vi "Disable Selected Opposing Channels.vi"(6 "Disabled? (False)":bool, 7 "Symbol Index (38)":i32=38, 8 "error in (no error)":errorcluster, 9 "Parent":string, 10 "Node Ptr":u64 format="%.0x", 11 "Tree":refnum<vi>) -> (0 "error out":errorcluster, 2 "Node Ptr":u64 format="%.0x", 3 "Tree Out":refnum<vi>)   [LabVIEW 2013, in "J1939 Addon System Explorer.lvlib"]
uses:
  J1939 Addon System Explorer.lvlib
  <vilib>/NI Veristand/Custom Device API/Custom Device API.lvlib
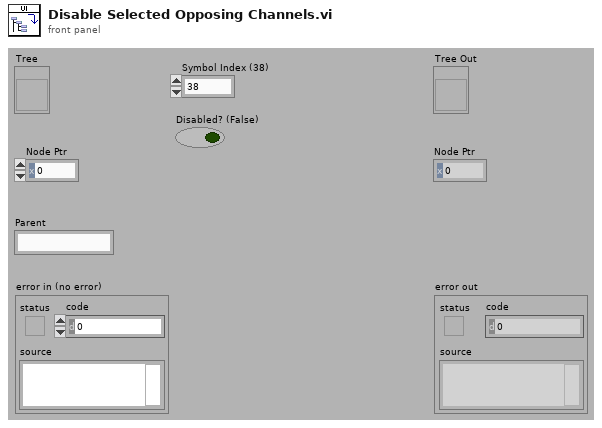
[diagram p1: front panel]
types:
  T1 = typedef "Custom Device API.lvlib/Custom Device Item Ref.ctl" = u64
  T2 = typedef "Custom Device API.lvlib/Custom Device Item Info.ctl" = cluster{"Name":string, "Is Channel":bool, "GUID":string, "Is Waveform":bool}
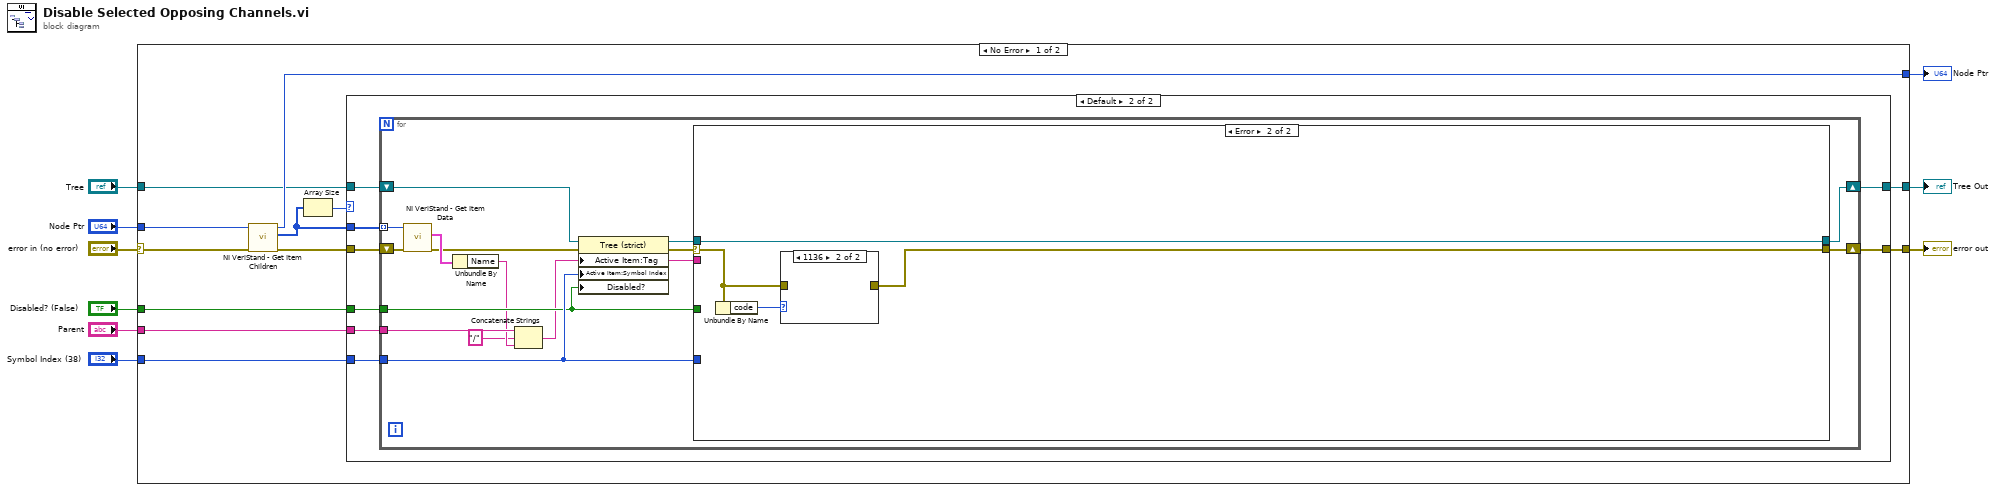
[diagram p0: block diagram]
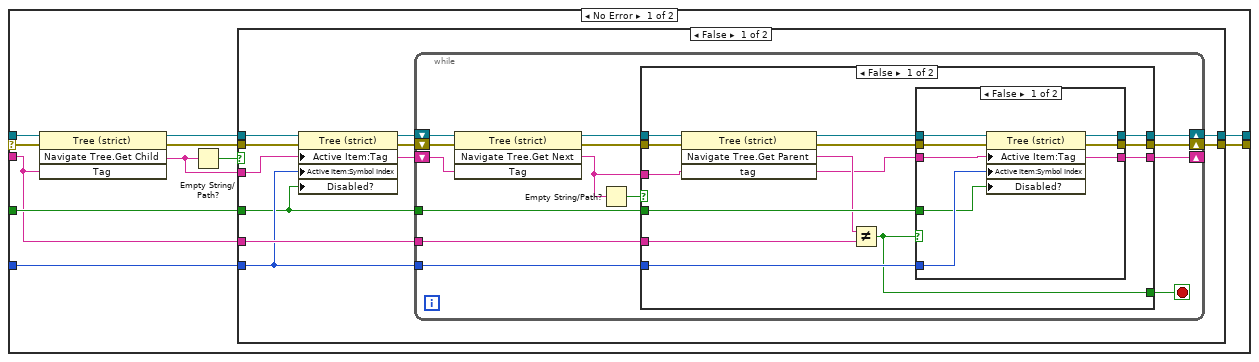
[diagram p3: hidden frame]
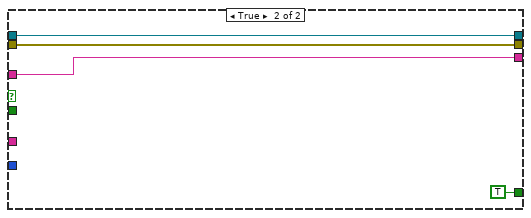
[diagram p5: hidden frame]
diagram:
  n1 = case shown="No Error" "error in (no error)" {
    selector: "error in (no error)" -> [w11 w118]
    tunnel: [w21 w118] -> w8
    tunnel: "Node Ptr" -> [w10 w116]
    tunnel: "Tree" -> [w17 w117]
    tunnel: [w20 w117] -> w5
    tunnel: "Parent" -> [w16 _]
    tunnel: [w19 w116] -> w3
    tunnel: "Symbol Index (38)" -> [w13 _]
    tunnel: "Disabled? (False)" -> [w12 _]
    frame No Error {
      n2 = call <vilib>:"NI VeriStand - Get Item Children.vi"("error in (no error)"=w11, "Item Ref in"=w10) -> ("error out"=w18:errorcluster, "Child Refs"=w15:T1[], "Item Ref out"=w19:T1)  [unwired: 6 in, 1 out]
      n3 = Array Size(array=w15) -> (size(s)=w14:i32)
      n4 = case shown="Default" w14 {
        tunnel: [w23 w31] -> w21
        tunnel: [w22 w30] -> w20
        tunnel: w18 -> [w23 w29]
        tunnel: w17 -> [w22 w28]
        tunnel: w16 -> [_ w26]
        tunnel: w15 -> [_ w25]
        tunnel: w13 -> [_ w24]
        tunnel: w12 -> [_ w27]
        frame 0 {
        }
        frame Default {
          n5 = for {
            tunnel: w25 -> [w45] mode=indexing
            shift-right: [w41] -> w30
            shift-left: w28 -> [w42]
            shift-right: [w40] -> w31
            shift-left: w29 -> [w46]
            tunnel: w26 -> [w39]
            tunnel: w24 -> [w38]
            tunnel: w27 -> [w37]
            n6 = call <vilib>:"NI VeriStand - Get Item Data.vi"("error in (no error)"=w46, "Item Ref in"=w45) -> ("error out"=w43:errorcluster, "Item Info"=w44:T2)  [unwired: 6 in, 2 out]
            n7 = Unbundle By Name(w44) -> ("Name"=w33:string)
            n8 = Concatenate Strings(w39, "/" ("string"), w33) -> (w34:string)
            n9 = property class="Tree (strict)"(reference=w42, error in=w43, "Active Item:Tag"=w34, "Active Item:Symbol Index"=w38, "Disabled?"=w37) -> (reference out=w36:refnum<vi>, error out=w35:errorcluster)
            n10 = case shown="Error" w35 {
              selector: w35 -> [w47 w111]
              tunnel: [w57 w114] -> w41
              tunnel: [w56 w112] -> w40
              tunnel: w38 -> [w55 _]
              tunnel: w37 -> [w54 _]
              tunnel: w34 -> [w53 _]
              tunnel: w36 -> [w52 w114]
              frame No Error {
                n11 = invoke class="Tree (strict)" method="Navigate Tree.Get Child"(reference=w52, error in=w47, "Tag"=w53) -> (reference out=w51:refnum<vi>, error out=w49:errorcluster, "Navigate Tree:Get Child"=w48:string)  [unwired: 1 in, 1 out]
                n12 = Empty String/Path?(string/path=w48) -> (empty?=w50:bool)
                n13 = case shown="False" w50 {
                  tunnel: [w67 w109] -> w57
                  tunnel: [w66 w110] -> w56
                  tunnel: w55 -> [w60 _]
                  tunnel: w54 -> [w59 _]
                  tunnel: w53 -> [w65 _]
                  tunnel: w51 -> [w62 w109]
                  tunnel: w49 -> [w64 w110]
                  tunnel: w48 -> [w58 _]
                  frame False {
                    n14 = property class="Tree (strict)"(reference=w62, error in=w64, "Active Item:Tag"=w58, "Active Item:Symbol Index"=w60, "Disabled?"=w59) -> (reference out=w61:refnum<vi>, error out=w63:errorcluster)
                    n15 = while {
                      shift-right: [w81] -> w67
                      shift-left: w61 -> [w77]
                      shift-right: [w80] -> w66
                      shift-left: w63 -> [w76]
                      tunnel: w65 -> [w72]
                      tunnel: w60 -> [w79]
                      tunnel: w59 -> [w78]
                      shift-right: [w71] -> _
                      shift-left: w58 -> [w75]
                      stop <- w70 stop-if-true
                      n16 = invoke class="Tree (strict)" method="Navigate Tree.Get Next"(reference=w77, error in=w76, "Tag"=w75) -> (reference out=w74:refnum<vi>, error out=w73:errorcluster, "Navigate Tree:Get Next Item"=w69:string)  [unwired: 1 in, 1 out]
                      n17 = Empty String/Path?(string/path=w69) -> (empty?=w68:bool)
                      n18 = case shown="False" w68 {
                        tunnel: [w94 w106] -> w81
                        tunnel: [w93 w107] -> w80
                        tunnel: w79 -> [w92 _]
                        tunnel: w78 -> [w91 _]
                        tunnel: w74 -> [w90 w106]
                        tunnel: w73 -> [w88 w107]
                        tunnel: w72 -> [w86 _]
                        tunnel: [w85 w108] -> w71
                        tunnel: [w84 TRUE] -> w70
                        tunnel: w69 -> [w82 w108]
                        frame False {
                          n19 = invoke class="Tree (strict)" method="Navigate Tree.Get Parent"(reference=w90, error in=w88, "tag"=w82) -> (reference out=w89:refnum<vi>, error out=w87:errorcluster, "Navigate Tree:Get Parent"=w83:string)  [unwired: 1 in, 1 out]
                          n20 = Not Equal?(x=w83, y=w86) -> (x != y?=w84:bool)
                          n21 = case shown="False" w84 {
                            tunnel: [w101 w102] -> w94
                            tunnel: [w100 w103] -> w93
                            tunnel: w92 -> [w99 _]
                            tunnel: w91 -> [w98 _]
                            tunnel: w89 -> [w97 w102]
                            tunnel: w87 -> [w96 w103]
                            tunnel: w82 -> [w95 w104]
                            tunnel: [w95 w104] -> w85
                            frame False {
                              n22 = property class="Tree (strict)"(reference=w97, error in=w96, "Active Item:Tag"=w95, "Active Item:Symbol Index"=w99, "Disabled?"=w98) -> (reference out=w101:refnum<vi>, error out=w100:errorcluster)
                            }
                            frame True {
                            }
                          }
                        }
                        frame True {
                        }
                      }
                    }
                  }
                  frame True {
                  }
                }
              }
              frame Error {
                n23 = Unbundle By Name(w111) -> ("code"=w113:i32)
                n24 = case shown="1136" w113 {
                  tunnel: [w115 _] -> w112
                  tunnel: w111 -> [w115 _]
                  frame Default {
                  }
                  frame 1136 {
                  }
                }
              }
            }
          }
        }
      }
    }
    frame Error {
    }
  }
  "error out" <- w8
  "Tree Out" <- w5
  "Node Ptr" <- w3
